vi "R3_Setup.vi"() -> (1 "tdms file out":refnum<k34>, 2 "error out":errorcluster)   [LabVIEW 2016]
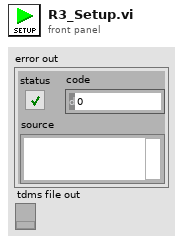
[diagram p1: front panel]
types:
  T1 = enum16{"open", "open or create", "create or replace", "create", "open (read-only)"}
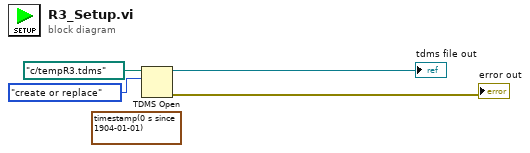
[diagram p0: block diagram]
diagram:
  (unwired) timestamp(0 s since 1904-01-01)
  n1 = TDMS Open(10:T1."create or replace" ("operation (0:open)"), 11:path "c:/tempR3.tdms" ("file path")) -> (0:→"error out":errorcluster, 3:→"tdms file out":refnum<k34>)  [unwired: 5 in]
